vi "Untitled 2.vi"   [LabVIEW 2015]
uses:
  Finite Acquisition - Solution/SubVIs/App Data.vi
types:
  T1 = typedef "Queue Data.ctl" = cluster{"Action":string}
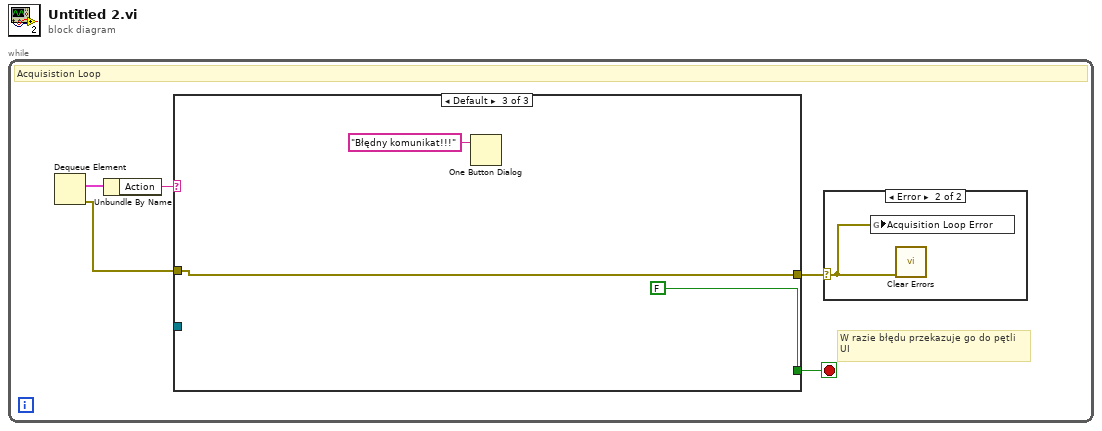
[diagram p0: block diagram]
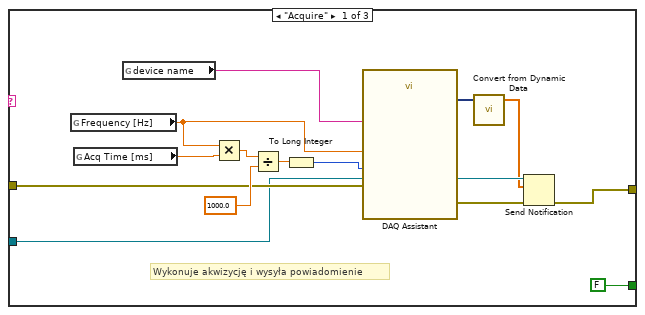
[diagram p3: hidden frame]
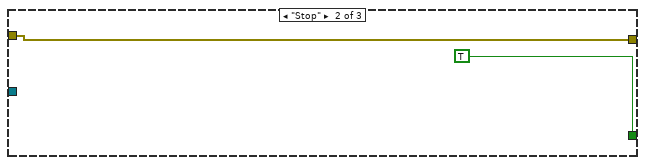
[diagram p4: hidden frame]
diagram:
  n1 = while {
    stop <- w2 stop-if-true
    # "W razie błędu przekazuje go do pętli\nUI"
    # "Acquisistion Loop"
    n2 = Dequeue Element() -> (element=w5:T1, error out=w3:errorcluster)  [unwired: 3 in, 2 out]
    n3 = Unbundle By Name(w5) -> ("Action"=w4:string)
    n4 = case shown="Default" w4 {
      tunnel: w3 -> [w14 w21 w24]
      tunnel: [FALSE TRUE FALSE] -> w2
      tunnel: [w10 w21 w24] -> w1
      tunnel: _ -> [w9 _ _]
      frame "Acquire" {
        # "Wykonuje akwizycję i wysyła powiadomienie"
        n5 = global read "App Data.vi" "Frequency [Hz]"() -> (w20:dbl)
        n6 = global read "App Data.vi" "Acq Time [ms]"() -> (w19:dbl)
        n7 = global read "App Data.vi" "device name"() -> (w12:tag)
        n8 = Multiply(x=w20, y=w19) -> (x*y=w18:dbl)
        n9 = Divide(x=w18, y=1000.0) -> (x/y=w16:dbl)
        n10 = To Long Integer(number=w16) -> (32bit integer=w15:i32)
        n11 = call "DAQ Assistant"("rate"=w20, "number of samples"=w15, "error in"=w14, "device name"=w12) -> ("data"=w8:dynamicdata, "error out"=w11:errorcluster)  [unwired: 13 in, 1 out]
        n12 = call "Convert from Dynamic Data"("Dynamic Data Type"=w8) -> ("Array"=w7:dbl[])  [unwired: 3 in]
        n13 = Send Notification(notification=w7, notifier=w9, error in (no error)=w11) -> (error out=w10:errorcluster)  [unwired: 1 out]
      }
      frame "Stop" {
      }
      frame Default {
        n14 = One Button Dialog(message="Błędny komunikat!!!") -> ()  [unwired: 1 in, 1 out]
      }
    }
    n15 = case shown="Error" w1 {
      selector: w1 -> [_ w6]
      frame No Error {
      }
      frame Error {
        n16 = global write "App Data.vi" "Acquisition Loop Error"(w6) -> ()
        n17 = call <vilib>:"Clear Errors.vi"("error in (no error)"=w6) -> ()  [unwired: 5 in, 2 out]
      }
    }
  }
